vi "ATE_BSE_Data Queue FGV.vi"(6 "Operations":T1, 8 "error in (no error)":errorcluster, 11 "Queue name":string) -> (0 "error out":errorcluster, 3 "queue out":refnum<queue>)   [LabVIEW 2021]
uses:
  Controls/ATE_BSE_Queue_Operations.ctl
  Controls/ATE_BSE_Controls_ref.ctl
  Controls/ATE_BSE_ref_type_Def.ctl
  SubVI's/IP Simulation/Controls/IP_Cellular Tech Type def.ctl
  SubVI's/IP Simulation/Controls/IP_Network_Type def.ctl
  SubVI's/IP Simulation/Controls/IP_Type-Tydedef.ctl
  SubVI's/Save File/Sim_Confi.ctl
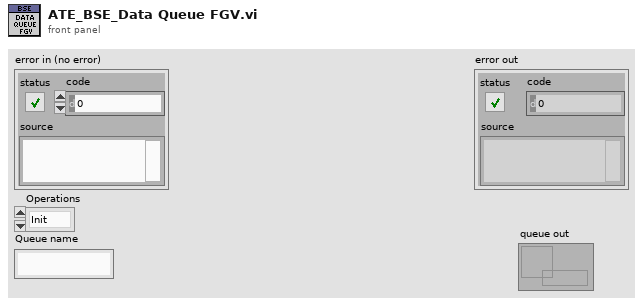
[diagram p1: front panel]
types:
  T1 = typedef "ATE_BSE_Queue_Operations.ctl" = enum16{"Init", "Get Queue", "Flush", "Close"}
  T2 = typedef "ATE_BSE_Controls_ref.ctl" = cluster{"Ref_Cluster":T3, "Time Stamp":timestamp, "Network-3":cluster{"NW3-Thr-Down":dbl, "NW3-Thr-Up":dbl, "NW3-Fre-Down":dbl, "NW3-Fre-Up":dbl, "NW3-PwL-Down":dbl, "NW3-PwL-Up":dbl}, "Network-2":cluster{"NW2-Thr-Down":dbl, "NW2-Thr-Up":dbl, "NW2-Fre-Down":dbl, "NW2-Fre-Up":dbl, "NW2-PwL-Down":dbl, "NW2-PwL-Up":dbl}, "Network-1":cluster{"NW1-Thr-Down":dbl, "NW1-Thr-Up":dbl, "NW1-Fre-Down":dbl, "NW1-Fre-Up":dbl, "NW1-PwL-Down":dbl, "NW1-PwL-Up":dbl}, "UE - 4":cluster{"UE4-Idle":bool, "UE4-Origination":bool, "UE4-Registration":bool, "UE4-Pdu Connection":bool, "UE4-Termination":bool, "UE4-Detach":bool}, "UE - 2":cluster{"UE2-Idle":bool, "UE2-Origination":bool, "UE2-Registration":bool, "UE2-Pdu Connection":bool, "UE2-Termination":bool, "UE2-Detach":bool}, "UE - 1":cluster{"UE1-Idle":bool, "UE1-Origination":bool, "UE1-Registration":bool, "UE1-Pdu Connection":bool, "UE1-Termination":bool, "UE1-Detach":bool}, "UE - 3":cluster{"UE3-Idle":bool, "UE3-Origination":bool, "UE3-Registration":bool, "UE3-Pdu Connection":bool, "UE3-Termination":bool, "UE3-Detach":bool}, "IP simulation":bool, "Start":bool, "Reset":bool, "Download":bool, "Upload":bool, "UE4":bool, "UE3":bool, "UE2":bool, "UE1":bool, "Trace_Table1":i32, "Status":string, "Trace_Table2":i32, "SelectNetwork1":cluster{"Nw1-check":bool, "NW-Combo":string}, "SelectNetwork2":cluster{"Nw1-check":bool, "NW-Combo":string}, "SelectNetwork3":cluster{"Nw1-check":bool, "NW-Combo":string}, "IMS":bool, "WWW":bool, "Sim Configuration":bool, "Ecall":bool, "Configurations":enum32{"Configurations", "Main"}, "Band":enum32{"GSM", "gNodeB", "eNodeB"}, "GSM-Data":enum32{"SDR", "CELL", "PHY", "GPRS"}, "eNodeB-Data":enum32{"SDR", "CELL", "PHY", "RRC"}, "gNodeB-Data":enum32{"SDR", "CELL", "PHY", "RRC"}, "Cancel Configurations":bool, "IP_UI":cluster{"Add":bool, "Close":bool, "IP_UI":cluster{"Cellular Tect":T4, "IP_NETWORK":T5, "IP_TYPE":T6, "IP_Client Address":string, "IP_ThgroughPut(Mbps)":i32, "Duration":i32, "Run":bool}[]}, "IMS_DATA":string[][], "ECall DATA":string[][], "Technology":string, "Sim Cluster in":T7, "Select BS":string, "Select Network 1":cluster{"Network 1-2G":cluster{"GSM-SDR":cluster{"DL Reference Power":i32, "Serail Name":string, "UL Reference Power":i32, "Radio Device":string}, "GSM-GPRS":cluster{"Priority Access THR":string, "Acess Burst Type":string, "Nack Countdown":string, "BCCH/PDCH Measurement":string, "Routing Area Code(RAC)":i32, "Network Control Order":string, "t3168":string, "t3192":string, "Alpha":string}, "GSM-PHY":cluster{"RACH Maximum Retransmission":string, "RACH Transmission Slots":string, "RACH Call Reestablishment":string, "RACH Access Control Class":string, "Block for Access Grant":string, "Multiframe for Paging":string, "Power Control Indicator":string, "Radio Link Timeout":string, "Cell Reselect Hysterisis":string, "Attach/Detach Allowed":string, "CCCH Combinations":string, "t3212":i64, "DTX Indicator":string, "Power Control Level":i64, "Minimum Received Signal Level":i64, "Half Rate Support":string, "Add Reselect":string}, "GSM-CELL":cluster{"SMS Enabled":string, "Eutra Operating Bands":string, "Power Offset Indicator":string, "Early Classmark Sending Control":string, "Location Area Code":i32, "CALL Enabled":string, "Loop Back Enabled":string, "GPRS Enabled":string, "SI Type 2 ter Indicator":string, "ARFCN":i64, "Frequency Format ID":i64, "Mobile Country Code":i64, "Mobile Network Code":i64, "Cell Barred Access":string, "Downlink Frequency":i32, "Uplink Frequency":i32}}, "Network 1-4G":cluster{"LTE-SDR":cluster{"Radio Device":string, "DL Reference Power":i32, "Serail Name":string, "UL Reference Power":i32, "DL Antennas":string, "UL Antennas":string}, "LTE-PHY":cluster{"PBCH Repetition":string, "PUCCH Delta Shift":string, "PUCCH CQI Number of RB":string, "PHICH Resource":string, "SRS Enable":string, "PCCH Paging Cycle":string, "BCCH Modification Coefficient":string, "PUSCH Alpha":string, "PUSCH DMRS Enable":string, "PHICH Duration":string, "PUCCH HARQ Max Transmission":i64, "PCCH Narrowband Count":string, "PUSCH Power Offset":i64, "PUCCH Power Offset":i64, "PDSCH Power Boost":string, "PUCCH An Occassions":string, "PUUCH CS Antenna Ports":string, "PRACH Response Window Size":string, "PRACH Contention Resolution Timer":string, "PRACH Ramping Step Size":string, "PDSCH Reference Power":i64, "PRACH Root Sequence Index":i64, "PRACH Maximum Transmissions":string, "PRACH Initial Received Target Power":string, "PRACH Configuration Index":i64}, "LTE-CELL":cluster{"Duplex Mode":string, "Measurement Report":string, "Eutra Operating Bands":string, "Carrier Bandwidth":string, "Physical Cell ID":i64, "Network Name":string, "DL Frequency":i32, "UL Frequency":i32, "Transmission Mode":string, "MNC Length":string, "IMS Enabled":string, "Tracking Area Code":i32, "Mobile Network Code":i32, "Mobile Country Code":i32}, "LTE-RRC":cluster{"RLC Maximum Retransmision Threshold":string, "RLC Timer Poll Retransmit":i32, "RLC Timer Reordering":i32, "RLC Timer Status Prohibit":i32, "RLC Poll PDU":i32, "RLC Poll Byte":i32}}, "Network 1-5G":cluster{"NR-SDR":cluster{"DL Reference Power":i32, "Serail Name":string, "UL Reference Power":i32, "DL Antennas":string, "UL Antennas":string, "Radio Device":string}, "NR-PHY":cluster{"PDSCH Reference Power":i64, "SSB RSRP Threshold":i64, "PRACH Contention Resolution Timer":i64, "Preamble Per SSB":i64, "Preamble Per SSB Format":i64, "UE Power Level Grant":i64, "RA Response Window":string, "Power Ramp Step Size":string, "Preamble Root Sequence Index":string, "Preamble Transmission Count":string, "Preamble Received Power":i64, "Zero Correlation Zone Configuration":i64, "Msg Frequency Division Multiplexing":string, "PRACH Configuration Index":i64, "Preamble Timing Offset":i64, "Preamble Format":i64, "Resource Restriction Type":string}, "NR-CELL":cluster{"Tracking Area Code":i64, "Mobile Country Code":i64, "Mobile Network Code":i64, "Operating Bands":string, "Physical Cell ID":i64, "DL Offset to Carrier":i32, "Subcarrier Spacing":string, "UL Offset to Carrier 2":i32, "Carrier Bandwidth":string, "Transmission Mode":string, "CSI-RS":string, "SRS":string, "Measurement Report":string}, "NR-RRC":cluster{"Ciphering Algorithms for SRB":string, "Integrity Algorithms for SRB":string, "Ciphering Algorithms for DRB":string, "Integrity Algorithms for DRB":string}}, "Technology-1":string}, "Select Network 2":cluster{"Network 2-2G":cluster{"GSM-SDR":cluster{"DL Reference Power":i32, "Serail Name":string, "UL Reference Power":i32, "Radio Device":string}, "GSM-GPRS":cluster{"Priority Access THR":string, "Acess Burst Type":string, "Nack Countdown":string, "BCCH/PDCH Measurement":string, "Routing Area Code(RAC)":i32, "Network Control Order":string, "t3168":string, "t3192":string, "Alpha":string}, "GSM-PHY":cluster{"RACH Maximum Retransmission":string, "RACH Transmission Slots":string, "RACH Call Reestablishment":string, "RACH Access Control Class":string, "Block for Access Grant":string, "Multiframe for Paging":string, "Power Control Indicator":string, "Radio Link Timeout":string, "Cell Reselect Hysterisis":string, "Attach/Detach Allowed":string, "CCCH Combinations":string, "t3212":i64, "DTX Indicator":string, "Power Control Level":i64, "Minimum Received Signal Level":i64, "Half Rate Support":string, "Add Reselect":string}, "GSM-CELL":cluster{"SMS Enabled":string, "Eutra Operating Bands":string, "Power Offset Indicator":string, "Early Classmark Sending Control":string, "Location Area Code":i32, "CALL Enabled":string, "Loop Back Enabled":string, "GPRS Enabled":string, "SI Type 2 ter Indicator":string, "ARFCN":i64, "Frequency Format ID":i64, "Mobile Country Code":i64, "Mobile Network Code":i64, "Cell Barred Access":string, "Downlink Frequency":i32, "Uplink Frequency":i32}}, "Network 2-4G":cluster{"LTE-SDR":cluster{"Radio Device":string, "DL Reference Power":i32, "Serail Name":string, "UL Reference Power":i32, "DL Antennas":string, "UL Antennas":string}, "LTE-PHY":cluster{"PBCH Repetition":string, "PUCCH Delta Shift":string, "PUCCH CQI Number of RB":string, "PHICH Resource":string, "SRS Enable":string, "PCCH Paging Cycle":string, "BCCH Modification Coefficient":string, "PUSCH Alpha":string, "PUSCH DMRS Enable":string, "PHICH Duration":string, "PUCCH HARQ Max Transmission":i64, "PCCH Narrowband Count":string, "PUSCH Power Offset":i64, "PUCCH Power Offset":i64, "PDSCH Power Boost":string, "PUCCH An Occassions":string, "PUUCH CS Antenna Ports":string, "PRACH Response Window Size":string, "PRACH Contention Resolution Timer":string, "PRACH Ramping Step Size":string, "PDSCH Reference Power":i64, "PRACH Root Sequence Index":i64, "PRACH Maximum Transmissions":string, "PRACH Initial Received Target Power":string, "PRACH Configuration Index":i64}, "LTE-CELL":cluster{"Duplex Mode":string, "Measurement Report":string, "Eutra Operating Bands":string, "Carrier Bandwidth":string, "Physical Cell ID":i64, "Network Name":string, "DL Frequency":i32, "UL Frequency":i32, "Transmission Mode":string, "MNC Length":string, "IMS Enabled":string, "Tracking Area Code":i32, "Mobile Network Code":i32, "Mobile Country Code":i32}, "LTE-RRC":cluster{"RLC Maximum Retransmision Threshold":string, "RLC Timer Poll Retransmit":i32, "RLC Timer Reordering":i32, "RLC Timer Status Prohibit":i32, "RLC Poll PDU":i32, "RLC Poll Byte":i32}}, "Network 2-5G":cluster{"NR-SDR":cluster{"DL Reference Power":i32, "Serail Name":string, "UL Reference Power":i32, "DL Antennas":string, "UL Antennas":string, "Radio Device":string}, "NR-PHY":cluster{"PDSCH Reference Power":i64, "SSB RSRP Threshold":i64, "PRACH Contention Resolution Timer":i64, "Preamble Per SSB":i64, "Preamble Per SSB Format":i64, "UE Power Level Grant":i64, "RA Response Window":string, "Power Ramp Step Size":string, "Preamble Root Sequence Index":string, "Preamble Transmission Count":string, "Preamble Received Power":i64, "Zero Correlation Zone Configuration":i64, "Msg Frequency Division Multiplexing":string, "PRACH Configuration Index":i64, "Preamble Timing Offset":i64, "Preamble Format":i64, "Resource Restriction Type":string}, "NR-CELL":cluster{"Tracking Area Code":i64, "Mobile Country Code":i64, "Mobile Network Code":i64, "Operating Bands":string, "Physical Cell ID":i64, "DL Offset to Carrier":i32, "Subcarrier Spacing":string, "UL Offset to Carrier 2":i32, "Carrier Bandwidth":string, "Transmission Mode":string, "CSI-RS":string, "SRS":string, "Measurement Report":string}, "NR-RRC":cluster{"Ciphering Algorithms for SRB":string, "Integrity Algorithms for SRB":string, "Ciphering Algorithms for DRB":string, "Integrity Algorithms for DRB":string}}, "Technology-2":string}, "Select Network 3":cluster{"Network 3-2G":cluster{"GSM-SDR":cluster{"DL Reference Power":i32, "Serail Name":string, "UL Reference Power":i32, "Radio Device":string}, "GSM-GPRS":cluster{"Priority Access THR":string, "Acess Burst Type":string, "Nack Countdown":string, "BCCH/PDCH Measurement":string, "Routing Area Code(RAC)":i32, "Network Control Order":string, "t3168":string, "t3192":string, "Alpha":string}, "GSM-PHY":cluster{"RACH Maximum Retransmission":string, "RACH Transmission Slots":string, "RACH Call Reestablishment":string, "RACH Access Control Class":string, "Block for Access Grant":string, "Multiframe for Paging":string, "Power Control Indicator":string, "Radio Link Timeout":string, "Cell Reselect Hysterisis":string, "Attach/Detach Allowed":string, "CCCH Combinations":string, "t3212":i64, "DTX Indicator":string, "Power Control Level":i64, "Minimum Received Signal Level":i64, "Half Rate Support":string, "Add Reselect":string}, "GSM-CELL":cluster{"SMS Enabled":string, "Eutra Operating Bands":string, "Power Offset Indicator":string, "Early Classmark Sending Control":string, "Location Area Code":i32, "CALL Enabled":string, "Loop Back Enabled":string, "GPRS Enabled":string, "SI Type 2 ter Indicator":string, "ARFCN":i64, "Frequency Format ID":i64, "Mobile Country Code":i64, "Mobile Network Code":i64, "Cell Barred Access":string, "Downlink Frequency":i32, "Uplink Frequency":i32}}, "Network 3-4G":cluster{"LTE-SDR":cluster{"Radio Device":string, "DL Reference Power":i32, "Serail Name":string, "UL Reference Power":i32, "DL Antennas":string, "UL Antennas":string}, "LTE-PHY":cluster{"PBCH Repetition":string, "PUCCH Delta Shift":string, "PUCCH CQI Number of RB":string, "PHICH Resource":string, "SRS Enable":string, "PCCH Paging Cycle":string, "BCCH Modification Coefficient":string, "PUSCH Alpha":string, "PUSCH DMRS Enable":string, "PHICH Duration":string, "PUCCH HARQ Max Transmission":i64, "PCCH Narrowband Count":string, "PUSCH Power Offset":i64, "PUCCH Power Offset":i64, "PDSCH Power Boost":string, "PUCCH An Occassions":string, "PUUCH CS Antenna Ports":string, "PRACH Response Window Size":string, "PRACH Contention Resolution Timer":string, "PRACH Ramping Step Size":string, "PDSCH Reference Power":i64, "PRACH Root Sequence Index":i64, "PRACH Maximum Transmissions":string, "PRACH Initial Received Target Power":string, "PRACH Configuration Index":i64}, "LTE-CELL":cluster{"Duplex Mode":string, "Measurement Report":string, "Eutra Operating Bands":string, "Carrier Bandwidth":string, "Physical Cell ID":i64, "Network Name":string, "DL Frequency":i32, "UL Frequency":i32, "Transmission Mode":string, "MNC Length":string, "IMS Enabled":string, "Tracking Area Code":i32, "Mobile Network Code":i32, "Mobile Country Code":i32}, "LTE-RRC":cluster{"RLC Maximum Retransmision Threshold":string, "RLC Timer Poll Retransmit":i32, "RLC Timer Reordering":i32, "RLC Timer Status Prohibit":i32, "RLC Poll PDU":i32, "RLC Poll Byte":i32}}, "Network 3-5G":cluster{"NR-SDR":cluster{"DL Reference Power":i32, "Serail Name":string, "UL Reference Power":i32, "DL Antennas":string, "UL Antennas":string, "Radio Device":string}, "NR-PHY":cluster{"PDSCH Reference Power":i64, "SSB RSRP Threshold":i64, "PRACH Contention Resolution Timer":i64, "Preamble Per SSB":i64, "Preamble Per SSB Format":i64, "UE Power Level Grant":i64, "RA Response Window":string, "Power Ramp Step Size":string, "Preamble Root Sequence Index":string, "Preamble Transmission Count":string, "Preamble Received Power":i64, "Zero Correlation Zone Configuration":i64, "Msg Frequency Division Multiplexing":string, "PRACH Configuration Index":i64, "Preamble Timing Offset":i64, "Preamble Format":i64, "Resource Restriction Type":string}, "NR-CELL":cluster{"Tracking Area Code":i64, "Mobile Country Code":i64, "Mobile Network Code":i64, "Operating Bands":string, "Physical Cell ID":i64, "DL Offset to Carrier":i32, "Subcarrier Spacing":string, "UL Offset to Carrier 2":i32, "Carrier Bandwidth":string, "Transmission Mode":string, "CSI-RS":string, "SRS":string, "Measurement Report":string}, "NR-RRC":cluster{"Ciphering Algorithms for SRB":string, "Integrity Algorithms for SRB":string, "Ciphering Algorithms for DRB":string, "Integrity Algorithms for DRB":string}}, "Technology-3":string}, "Current Technology":string, "Current Network":string}
  T3 = typedef "ATE_BSE_ref_type_Def.ctl" = cluster{"UE1":refnum<vi>, "UE2":refnum<vi>, "UE3":refnum<vi>, "SelectNetwork1":refnum<vi>, "SelectNetwork3":refnum<vi>, "SelectNetwork2":refnum<vi>, "Trace_Table1":refnum<vi>, "UE - 1":refnum<vi>, "UE - 2":refnum<vi>, "UE - 3":refnum<vi>, "UE - 4":refnum<vi>, "Network-3":refnum<vi>, "Status":refnum<vi>, "Trace_Table2":refnum<vi>, "UE4":refnum<vi>, "Start":refnum<vi>, "Reset":refnum<vi>, "IP simulation":refnum<vi>, "Network-1":refnum<vi>, "Time Stamp":refnum<vi>, "Network-2":refnum<vi>, "IMS":refnum<vi>, "GSM-Data":refnum<vi>, "Configurations":refnum<vi>, "Band":refnum<vi>, "Sim Configurations":refnum<vi>, "ECall":refnum<vi>, "WWW":refnum<vi>, "Cancel Configurations":refnum<vi>, "GSM-PHY":refnum<vi>, "GSM-CELL":refnum<vi>, "GSM-GPRS":refnum<vi>, "LTE-CELL":refnum<vi>, "LTE-PHY":refnum<vi>, "LTE-RRC":refnum<vi>, "LTE-SDR":refnum<vi>, "NR-RRC":refnum<vi>, "NR-SDR":refnum<vi>, "NR-PHY":refnum<vi>, "NR-CELL":refnum<vi>, "GSM-SDR":refnum<vi>, "gNodeB-Data":refnum<vi>, "eNodeB-Data":refnum<vi>, "Select BS":refnum<vi>, "Download":refnum<vi>, "Upload":refnum<vi>}
  T4 = typedef "IP_Cellular Tech Type def.ctl" = string
  T5 = typedef "IP_Network_Type def.ctl" = string
  T6 = typedef "IP_Type-Tydedef.ctl" = string
  T7 = typedef "Sim_Confi.ctl" = cluster{"Session_array":cluster{"Add Bearer":bool, "APN Name\n":string, "AMBR Uplink(Gbps)\n":string, "AMBR Downlink(Gbps)\n":string, "Session name":string, "Bearer_Array":cluster{"QCI:":string, "Priority Level:":string, "Pre-emption\nCapability:":string, "Pre-emption\nVulnerability:":string, "MBR DL:":string, "MBR UL:":string, "GBR DL:":string, "GBR UL:":string, "Bearer Name":string, "Delete Session":bool}[], "Delete Session":bool}[], "SIM_U_Config":cluster{"Add":bool, "Close":bool, "SIM_UI":cluster{"Delete":bool, "Edit":bool, "TAC":string, "OP Value":string, "K Value":string, "Phone Number":string, "IMSI":string}[], "Save":bool}}
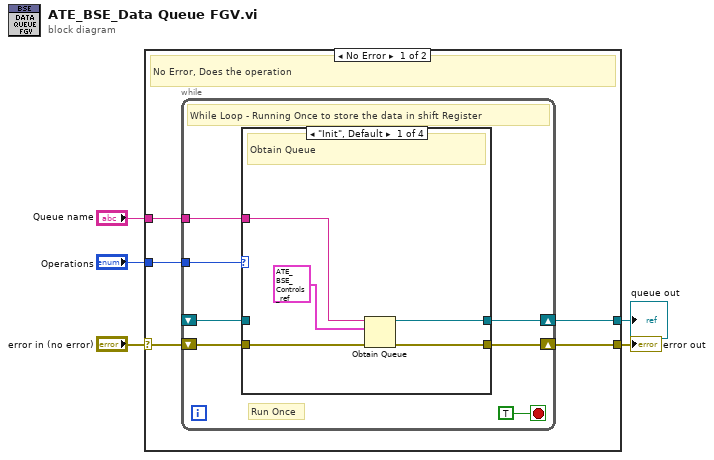
[diagram p0: block diagram]
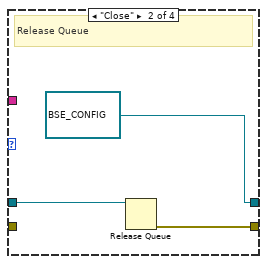
[diagram p2: hidden frame]
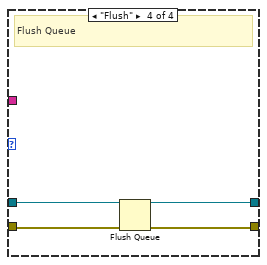
[diagram p4: hidden frame]
diagram:
  n1 = case shown="No Error" "error in (no error)" {
    selector: "error in (no error)" -> [w9 w32]
    tunnel: [w8 w32] -> w2
    tunnel: "Operations" -> [w10 _]
    tunnel: "Queue name" -> [w7 _]
    tunnel: [w6 _] -> w1
    frame No Error {
      # "No Error, Does the operation"
      n2 = while {
        tunnel: w10 -> [w16]
        shift-right: [w14] -> w8
        shift-left: w9 -> [w15]
        tunnel: w7 -> [w13]
        shift-right: [w12] -> w6
        shift-left: _ -> [w11]
        stop <- TRUE stop-if-true
        # "Run Once"
        # "While Loop - Running Once to store the data in shift Register"
        n3 = case shown="\"Init\", Default" w16 {
          tunnel: w15 -> [w22 _ w26 w30]
          tunnel: [w21 w24 w26 w29] -> w14
          tunnel: w13 -> [w20 _ _ _]
          tunnel: [w19 refnum<queue> refnum ("queue out") w27 w28] -> w12
          tunnel: w11 -> [_ w25 w27 w31]
          frame "Init", Default {
            # "Obtain Queue"
            n4 = Obtain Queue(name (unnamed)=w20, element data type=T2 {"Ref_Cluster"={"UE1"=refnum, "UE2"=refnum, "UE3"=refnum, "SelectNetwork1"=refnum, "SelectNetwork3"=refnum, "SelectNetwork2"=refnum, "Trace_Table1"=refnum, "UE - 1"=refnum, "UE - 2"=refnum, "UE - 3"=refnum, "UE - 4"=refnum, "Network-3"=refnum, "Status"=refnum, "Trace_Table2"=refnum, "UE4"=refnum, "Start"=refnum, "Reset"=refnum, "IP simulation"=refnum, "Network-1"=refnum, "Time Stamp"=refnum, "Network-2"=refnum, "IMS"=refnum, "GSM-Data"=refnum, "Configurations"=refnum, "Band"=refnum, "Sim Configurations"=refnum, "ECall"=refnum, "WWW"=refnum, "Cancel Configurations"=refnum, "GSM-PHY"=refnum, "GSM-CELL"=refnum, "GSM-GPRS"=refnum, "LTE-CELL"=refnum, "LTE-PHY"=refnum, "LTE-RRC"=refnum, "LTE-SDR"=refnum, "NR-RRC"=refnum, "NR-SDR"=refnum, "NR-PHY"=refnum, "NR-CELL"=refnum, "GSM-SDR"=refnum, "gNodeB-Data"=refnum, "eNodeB-Data"=refnum, "Select BS"=refnum, "Download"=refnum, "Upload"=refnum}, "Time Stamp"=timestamp(0 s since 1904-01-01), "Network-3"={"NW3-Thr-Down"=0.0, "NW3-Thr-Up"=0.0, "NW3-Fre-Down"=0.0, "NW3-Fre-Up"=0.0, "NW3-PwL-Down"=0.0, "NW3-PwL-Up"=0.0}, "Network-2"={"NW2-Thr-Down"=0.0, "NW2-Thr-Up"=0.0, "NW2-Fre-Down"=0.0, "NW2-Fre-Up"=0.0, "NW2-PwL-Down"=0.0, "NW2-PwL-Up"=0.0}, "Network-1"={"NW1-Thr-Down"=0.0, "NW1-Thr-Up"=0.0, "NW1-Fre-Down"=0.0, "NW1-Fre-Up"=0.0, "NW1-PwL-Down"=0.0, "NW1-PwL-Up"=0.0}, "UE - 4"={"UE4-Idle"=FALSE, "UE4-Origination"=FALSE, "UE4-Registration"=FALSE, "UE4-Pdu Connection"=FALSE, "UE4-Termination"=FALSE, "UE4-Detach"=FALSE}, "UE - 2"={"UE2-Idle"=FALSE, "UE2-Origination"=FALSE, "UE2-Registration"=FALSE, "UE2-Pdu Connection"=FALSE, "UE2-Termination"=FALSE, "UE2-Detach"=FALSE}, "UE - 1"={"UE1-Idle"=FALSE, "UE1-Origination"=FALSE, "UE1-Registration"=FALSE, "UE1-Pdu Connection"=FALSE, "UE1-Termination"=FALSE, "UE1-Detach"=FALSE}, "UE - 3"={"UE3-Idle"=FALSE, "UE3-Origination"=FALSE, "UE3-Registration"=FALSE, "UE3-Pdu Connection"=FALSE, "UE3-Termination"=FALSE, "UE3-Detach"=FALSE}, "IP simulation"=FALSE, "Start"=FALSE, "Reset"=FALSE, "Download"=FALSE, "Upload"=FALSE, "UE4"=FALSE, "UE3"=FALSE, "UE2"=FALSE, "UE1"=FALSE, "Trace_Table1"=0, "Status"="", "Trace_Table2"=0, "SelectNetwork1"={"Nw1-check"=FALSE, "NW-Combo"="GSM"}, "SelectNetwork2"={"Nw1-check"=FALSE, "NW-Combo"="GSM"}, "SelectNetwork3"={"Nw1-check"=FALSE, "NW-Combo"="GSM"}, "IMS"=FALSE, "WWW"=FALSE, "Sim Configuration"=FALSE, "Ecall"=FALSE, "Configurations"=enum."Configurations", "Band"=enum."GSM", "GSM-Data"=enum."SDR", "eNodeB-Data"=enum."RRC", "gNodeB-Data"=enum."SDR", "Cancel Configurations"=FALSE, "IP_UI"={"Add"=FALSE, "Close"=FALSE, "IP_UI"=[]}, "IMS_DATA"=[], "ECall DATA"=[], "Technology"="", "Sim Cluster in"={"Session_array"=[{"Add Bearer"=FALSE, "APN Name\n"="as", "AMBR Uplink(Gbps)\n"="as", "AMBR Downlink(Gbps)\n"="11111111111111111111111111111111", "Session name"="8baf473f2f8fd09487cccbd7097c6862", "Bearer_Array"=[], "Delete Session"=FALSE}], "SIM_U_Config"={"Add"=FALSE, "Close"=TRUE, "SIM_UI"=[], "Save"=FALSE}}, "Select BS"="", "Select Network 1"={"Network 1-2G"={"GSM-SDR"={"DL Reference Power"=-13, "Serail Name"="", "UL Reference Power"=-13, "Radio Device"="0"}, "GSM-GPRS"={"Priority Access THR"="6", "Acess Burst Type"="0", "Nack Countdown"="8", "BCCH/PDCH Measurement"="0", "Routing Area Code(RAC)"=128, "Network Control Order"="0", "t3168"="3", "t3192"="2", "Alpha"="10"}, "GSM-PHY"={"RACH Maximum Retransmission"="3", "RACH Transmission Slots"="1", "RACH Call Reestablishment"="1", "RACH Access Control Class"="1", "Block for Access Grant"="0", "Multiframe for Paging"="0", "Power Control Indicator"="0", "Radio Link Timeout"="850", "Cell Reselect Hysterisis"="0", "Attach/Detach Allowed"="0", "CCCH Combinations"="0", "t3212"=0, "DTX Indicator"="1", "Power Control Level"=0, "Minimum Received Signal Level"=0, "Half Rate Support"="0", "Add Reselect"="1"}, "GSM-CELL"={"SMS Enabled"="0", "Eutra Operating Bands"="3", "Power Offset Indicator"="", "Early Classmark Sending Control"="1", "Location Area Code"=0, "CALL Enabled"="1", "Loop Back Enabled"="0", "GPRS Enabled"="1", "SI Type 2 ter Indicator"="0", "ARFCN"=1, "Frequency Format ID"=1, "Mobile Country Code"=1, "Mobile Network Code"=1, "Cell Barred Access"="ONESIXTH", "Downlink Frequency"=-13, "Uplink Frequency"=1842}}, "Network 1-4G"={"LTE-SDR"={"Radio Device"="0", "DL Reference Power"=-13, "Serail Name"="", "UL Reference Power"=-13, "DL Antennas"="1", "UL Antennas"="1"}, "LTE-PHY"={"PBCH Repetition"="0", "PUCCH Delta Shift"="0", "PUCCH CQI Number of RB"="2", "PHICH Resource"="0", "SRS Enable"="0", "PCCH Paging Cycle"="1", "BCCH Modification Coefficient"="10", "PUSCH Alpha"="48", "PUSCH DMRS Enable"="4", "PHICH Duration"="10", "PUCCH HARQ Max Transmission"=-27, "PCCH Narrowband Count"="-108", "PUSCH Power Offset"=0, "PUCCH Power Offset"=0, "PDSCH Power Boost"="0", "PUCCH An Occassions"="1", "PUUCH CS Antenna Ports"="10", "PRACH Response Window Size"="MaxEye", "PRACH Contention Resolution Timer"="TM1", "PRACH Ramping Step Size"="2", "PDSCH Reference Power"=-27, "PRACH Root Sequence Index"=80, "PRACH Maximum Transmissions"="0", "PRACH Initial Received Target Power"="4", "PRACH Configuration Index"=98}, "LTE-CELL"={"Duplex Mode"="10", "Measurement Report"="1", "Eutra Operating Bands"="139", "Carrier Bandwidth"="10", "Physical Cell ID"=0, "Network Name"="one", "DL Frequency"=4, "UL Frequency"=25, "Transmission Mode"="TM1", "MNC Length"="77", "IMS Enabled"="1", "Tracking Area Code"=1, "Mobile Network Code"=1, "Mobile Country Code"=1}, "LTE-RRC"={"RLC Maximum Retransmision Threshold"="1", "RLC Timer Poll Retransmit"=0, "RLC Timer Reordering"=0, "RLC Timer Status Prohibit"=-96, "RLC Poll PDU"=13, "RLC Poll Byte"=1}}, "Network 1-5G"={"NR-SDR"={"DL Reference Power"=0, "Serail Name"="1", "UL Reference Power"=-13, "DL Antennas"="0", "UL Antennas"="0", "Radio Device"="1"}, "NR-PHY"={"PDSCH Reference Power"=-27, "SSB RSRP Threshold"=-109, "PRACH Contention Resolution Timer"=7, "Preamble Per SSB"=14, "Preamble Per SSB Format"=4, "UE Power Level Grant"=-90, "RA Response Window"="1", "Power Ramp Step Size"="2", "Preamble Root Sequence Index"="139", "Preamble Transmission Count"="10", "Preamble Received Power"=-96, "Zero Correlation Zone Configuration"=13, "Msg Frequency Division Multiplexing"="one", "PRACH Configuration Index"=98, "Preamble Timing Offset"=1, "Preamble Format"=0, "Resource Restriction Type"="0"}, "NR-CELL"={"Tracking Area Code"=1, "Mobile Country Code"=1, "Mobile Network Code"=1, "Operating Bands"="77", "Physical Cell ID"=0, "DL Offset to Carrier"=0, "Subcarrier Spacing"="1", "UL Offset to Carrier 2"=0, "Carrier Bandwidth"="10", "Transmission Mode"="TM1", "CSI-RS"="1", "SRS"="1", "Measurement Report"="1"}, "NR-RRC"={"Ciphering Algorithms for SRB"="0", "Integrity Algorithms for SRB"="0", "Ciphering Algorithms for DRB"="1", "Integrity Algorithms for DRB"="1"}}, "Technology-1"=""}, "Select Network 2"={"Network 2-2G"={"GSM-SDR"={"DL Reference Power"=-13, "Serail Name"="", "UL Reference Power"=-13, "Radio Device"="0"}, "GSM-GPRS"={"Priority Access THR"="6", "Acess Burst Type"="0", "Nack Countdown"="8", "BCCH/PDCH Measurement"="0", "Routing Area Code(RAC)"=128, "Network Control Order"="0", "t3168"="3", "t3192"="2", "Alpha"="10"}, "GSM-PHY"={"RACH Maximum Retransmission"="1", "RACH Transmission Slots"="14", "RACH Call Reestablishment"="1", "RACH Access Control Class"="0", "Block for Access Grant"="2", "Multiframe for Paging"="0", "Power Control Indicator"="0", "Radio Link Timeout"="15", "Cell Reselect Hysterisis"="3", "Attach/Detach Allowed"="1", "CCCH Combinations"="1", "t3212"=0, "DTX Indicator"="1", "Power Control Level"=0, "Minimum Received Signal Level"=0, "Half Rate Support"="0", "Add Reselect"="0"}, "GSM-CELL"={"SMS Enabled"="0", "Eutra Operating Bands"="850", "Power Offset Indicator"="0", "Early Classmark Sending Control"="0", "Location Area Code"=1, "CALL Enabled"="0", "Loop Back Enabled"="1", "GPRS Enabled"="0", "SI Type 2 ter Indicator"="1", "ARFCN"=0, "Frequency Format ID"=71, "Mobile Country Code"=1, "Mobile Network Code"=1, "Cell Barred Access"="0", "Downlink Frequency"=0, "Uplink Frequency"=900200000}}, "Network 2-4G"={"LTE-SDR"={"Radio Device"="0", "DL Reference Power"=-13, "Serail Name"="", "UL Reference Power"=-13, "DL Antennas"="1", "UL Antennas"="1"}, "LTE-PHY"={"PBCH Repetition"="0", "PUCCH Delta Shift"="1", "PUCCH CQI Number of RB"="0", "PHICH Resource"="ONESIXTH", "SRS Enable"="0", "PCCH Paging Cycle"="256", "BCCH Modification Coefficient"="2", "PUSCH Alpha"="1", "PUSCH DMRS Enable"="0", "PHICH Duration"="0", "PUCCH HARQ Max Transmission"=4, "PCCH Narrowband Count"="2", "PUSCH Power Offset"=-96, "PUCCH Power Offset"=-96, "PDSCH Power Boost"="0", "PUCCH An Occassions"="0", "PUUCH CS Antenna Ports"="1", "PRACH Response Window Size"="10", "PRACH Contention Resolution Timer"="48", "PRACH Ramping Step Size"="4", "PDSCH Reference Power"=-27, "PRACH Root Sequence Index"=0, "PRACH Maximum Transmissions"="10", "PRACH Initial Received Target Power"="-108", "PRACH Configuration Index"=0}, "LTE-CELL"={"Duplex Mode"="0", "Measurement Report"="1", "Eutra Operating Bands"="3", "Carrier Bandwidth"="10", "Physical Cell ID"=0, "Network Name"="MaxEye", "DL Frequency"=1842, "UL Frequency"=1747, "Transmission Mode"="TM1", "MNC Length"="2", "IMS Enabled"="0", "Tracking Area Code"=1, "Mobile Network Code"=1, "Mobile Country Code"=1}, "LTE-RRC"={"RLC Maximum Retransmision Threshold"="4", "RLC Timer Poll Retransmit"=80, "RLC Timer Reordering"=35, "RLC Timer Status Prohibit"=0, "RLC Poll PDU"=4, "RLC Poll Byte"=25}}, "Network 2-5G"={"NR-SDR"={"DL Reference Power"=-13, "Serail Name"="", "UL Reference Power"=-13, "DL Antennas"="1", "UL Antennas"="1", "Radio Device"="0"}, "NR-PHY"={"PDSCH Reference Power"=-27, "SSB RSRP Threshold"=-109, "PRACH Contention Resolution Timer"=7, "Preamble Per SSB"=14, "Preamble Per SSB Format"=4, "UE Power Level Grant"=-90, "RA Response Window"="10", "Power Ramp Step Size"="2", "Preamble Root Sequence Index"="139", "Preamble Transmission Count"="10", "Preamble Received Power"=-96, "Zero Correlation Zone Configuration"=13, "Msg Frequency Division Multiplexing"="one", "PRACH Configuration Index"=98, "Preamble Timing Offset"=1, "Preamble Format"=0, "Resource Restriction Type"="0"}, "NR-CELL"={"Tracking Area Code"=1, "Mobile Country Code"=1, "Mobile Network Code"=1, "Operating Bands"="77", "Physical Cell ID"=0, "DL Offset to Carrier"=0, "Subcarrier Spacing"="1", "UL Offset to Carrier 2"=0, "Carrier Bandwidth"="10", "Transmission Mode"="TM1", "CSI-RS"="1", "SRS"="1", "Measurement Report"="1"}, "NR-RRC"={"Ciphering Algorithms for SRB"="0", "Integrity Algorithms for SRB"="0", "Ciphering Algorithms for DRB"="1", "Integrity Algorithms for DRB"="1"}}, "Technology-2"=""}, "Select Network 3"={"Network 3-2G"={"GSM-SDR"={"DL Reference Power"=-13, "Serail Name"="", "UL Reference Power"=-13, "Radio Device"="0"}, "GSM-GPRS"={"Priority Access THR"="6", "Acess Burst Type"="0", "Nack Countdown"="8", "BCCH/PDCH Measurement"="0", "Routing Area Code(RAC)"=128, "Network Control Order"="0", "t3168"="3", "t3192"="2", "Alpha"="10"}, "GSM-PHY"={"RACH Maximum Retransmission"="1", "RACH Transmission Slots"="14", "RACH Call Reestablishment"="1", "RACH Access Control Class"="0", "Block for Access Grant"="2", "Multiframe for Paging"="0", "Power Control Indicator"="0", "Radio Link Timeout"="15", "Cell Reselect Hysterisis"="3", "Attach/Detach Allowed"="1", "CCCH Combinations"="1", "t3212"=0, "DTX Indicator"="1", "Power Control Level"=0, "Minimum Received Signal Level"=0, "Half Rate Support"="0", "Add Reselect"="0"}, "GSM-CELL"={"SMS Enabled"="0", "Eutra Operating Bands"="850", "Power Offset Indicator"="0", "Early Classmark Sending Control"="0", "Location Area Code"=1, "CALL Enabled"="0", "Loop Back Enabled"="1", "GPRS Enabled"="0", "SI Type 2 ter Indicator"="1", "ARFCN"=0, "Frequency Format ID"=71, "Mobile Country Code"=1, "Mobile Network Code"=1, "Cell Barred Access"="0", "Downlink Frequency"=0, "Uplink Frequency"=900200000}}, "Network 3-4G"={"LTE-SDR"={"Radio Device"="0", "DL Reference Power"=-13, "Serail Name"="", "UL Reference Power"=-13, "DL Antennas"="1", "UL Antennas"="1"}, "LTE-PHY"={"PBCH Repetition"="0", "PUCCH Delta Shift"="1", "PUCCH CQI Number of RB"="0", "PHICH Resource"="ONESIXTH", "SRS Enable"="0", "PCCH Paging Cycle"="256", "BCCH Modification Coefficient"="2", "PUSCH Alpha"="1", "PUSCH DMRS Enable"="0", "PHICH Duration"="0", "PUCCH HARQ Max Transmission"=4, "PCCH Narrowband Count"="2", "PUSCH Power Offset"=-96, "PUCCH Power Offset"=-96, "PDSCH Power Boost"="0", "PUCCH An Occassions"="0", "PUUCH CS Antenna Ports"="1", "PRACH Response Window Size"="10", "PRACH Contention Resolution Timer"="48", "PRACH Ramping Step Size"="4", "PDSCH Reference Power"=-27, "PRACH Root Sequence Index"=0, "PRACH Maximum Transmissions"="10", "PRACH Initial Received Target Power"="-108", "PRACH Configuration Index"=0}, "LTE-CELL"={"Duplex Mode"="0", "Measurement Report"="1", "Eutra Operating Bands"="3", "Carrier Bandwidth"="10", "Physical Cell ID"=0, "Network Name"="MaxEye", "DL Frequency"=1842, "UL Frequency"=1747, "Transmission Mode"="TM1", "MNC Length"="2", "IMS Enabled"="0", "Tracking Area Code"=1, "Mobile Network Code"=1, "Mobile Country Code"=1}, "LTE-RRC"={"RLC Maximum Retransmision Threshold"="4", "RLC Timer Poll Retransmit"=80, "RLC Timer Reordering"=35, "RLC Timer Status Prohibit"=0, "RLC Poll PDU"=4, "RLC Poll Byte"=25}}, "Network 3-5G"={"NR-SDR"={"DL Reference Power"=-13, "Serail Name"="", "UL Reference Power"=-13, "DL Antennas"="1", "UL Antennas"="1", "Radio Device"="0"}, "NR-PHY"={"PDSCH Reference Power"=-27, "SSB RSRP Threshold"=-109, "PRACH Contention Resolution Timer"=7, "Preamble Per SSB"=14, "Preamble Per SSB Format"=4, "UE Power Level Grant"=-90, "RA Response Window"="10", "Power Ramp Step Size"="2", "Preamble Root Sequence Index"="139", "Preamble Transmission Count"="10", "Preamble Received Power"=-96, "Zero Correlation Zone Configuration"=13, "Msg Frequency Division Multiplexing"="one", "PRACH Configuration Index"=98, "Preamble Timing Offset"=1, "Preamble Format"=0, "Resource Restriction Type"="0"}, "NR-CELL"={"Tracking Area Code"=1, "Mobile Country Code"=1, "Mobile Network Code"=1, "Operating Bands"="77", "Physical Cell ID"=0, "DL Offset to Carrier"=0, "Subcarrier Spacing"="1", "UL Offset to Carrier 2"=0, "Carrier Bandwidth"="10", "Transmission Mode"="TM1", "CSI-RS"="1", "SRS"="1", "Measurement Report"="1"}, "NR-RRC"={"Ciphering Algorithms for SRB"="0", "Integrity Algorithms for SRB"="0", "Ciphering Algorithms for DRB"="1", "Integrity Algorithms for DRB"="1"}}, "Technology-3"=""}, "Current Technology"="", "Current Network"=""} ("BSE_CONFIG"), error in (no error)=w22) -> (queue out=w19:refnum<queue>, error out=w21:errorcluster)  [unwired: 2 in, 1 out]
          }
          frame "Close" {
            # "Release Queue"
            n5 = Release Queue(queue=w25) -> (error out=w24:errorcluster)  [unwired: 2 in, 2 out]
          }
          frame "Get Queue" {
            # "Enqueue the Element into the Queue"
          }
          frame "Flush" {
            # "Flush Queue"
            n6 = Flush Queue(queue=w31, error in (no error)=w30) -> (queue out=w28:refnum<queue>, error out=w29:errorcluster)  [unwired: 1 out]
          }
        }
      }
    }
    frame Error {
      # "Gives out the next state as Error"
      # "Error, Does nothing"
    }
  }
  "error out" <- w2
  "queue out" <- w1
